vi "Write val.vi"(8 "error in (no error)":errorcluster, 10 "val":u8, 11 "PowerSupply MSG in":refnum<class "PowerSupply MSG.lvclass">) -> (0 "error out":errorcluster, 3 "PowerSupply MSG out":refnum<class "PowerSupply MSG.lvclass">)   [LabVIEW 2014, in "Controller.lvlib" / "PowerSupply MSG.lvclass"]
uses:
  PowerSupply MSG.lvclass
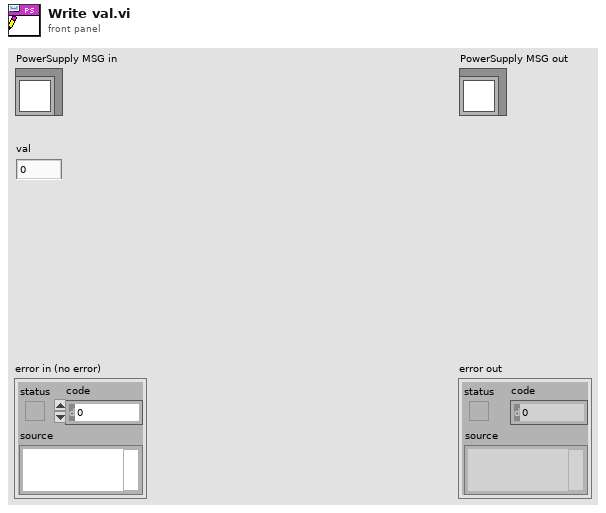
[diagram p1: front panel]
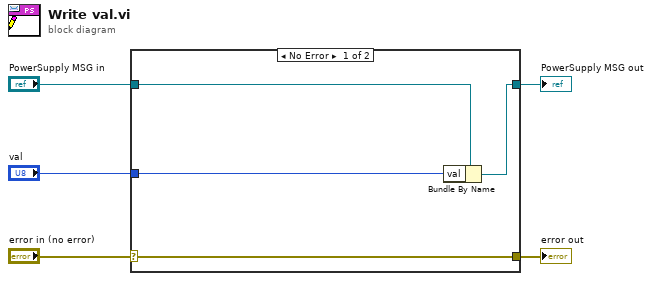
[diagram p0: block diagram]
diagram:
  n1 = case shown="No Error" "error in (no error)" {
    selector: "error in (no error)" -> [w9 w10]
    tunnel: [w9 w10] -> w4
    tunnel: [w7 w11] -> w2
    tunnel: "PowerSupply MSG in" -> [w8 w11]
    tunnel: "val" -> [w6 _]
    frame No Error {
      n2 = Bundle By Name(cluster=w8, "val"=w6) -> (w7:refnum<class "PowerSupply MSG.lvclass">)
    }
    frame Error {
    }
  }
  "error out" <- w4
  "PowerSupply MSG out" <- w2
